vi "CompressAndUpdate(Enum).vi"(7 "force CVT update (false)":bool, 8 "error in":errorcluster, 9 "precision (6)":i16=6, 10 "enum variant":variant, 11 "command or variable name":string) -> (0 "error out":errorcluster)   [LabVIEW 2011]
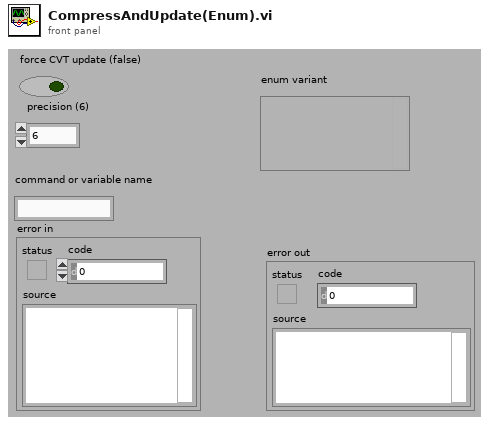
[diagram p1: front panel]
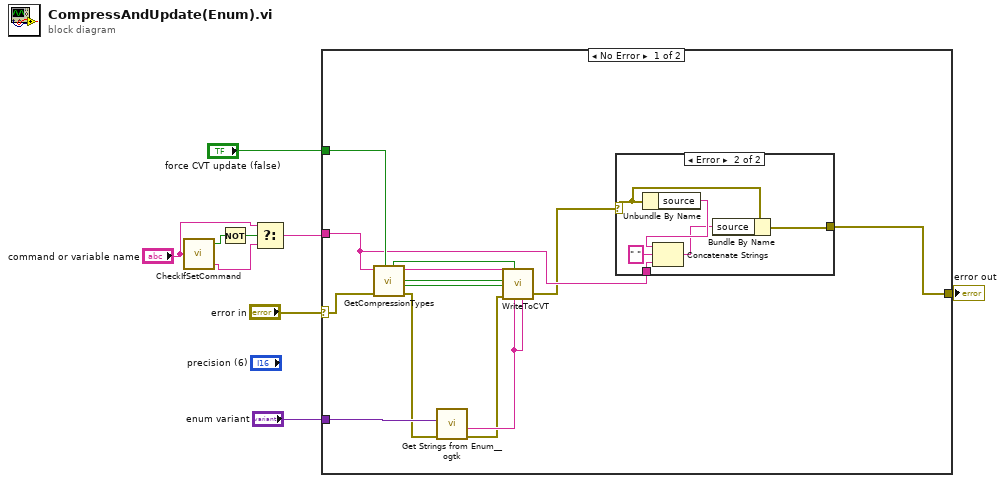
[diagram p0: block diagram]
diagram:
  n1 = call "CheckIfSetCommand.vi"("Command"="command or variable name") -> ("setCommand?"=w7:bool, "variable"=w4:string)  [unwired: 1 out]
  n2 = Not(x=w7) -> (.not. x?=w6:bool)
  n3 = Select(t="command or variable name", s=w6, f=w4) -> (s? t:f=w3:string)
  n4 = case shown="No Error" "error in" {
    selector: "error in" -> [w21 w30]
    tunnel: w3 -> [w12 _]
    tunnel: [w10 w30] -> w8
    tunnel: "force CVT update (false)" -> [w13 _]
    tunnel: "enum variant" -> [w22 _]
    frame No Error {
      n5 = call "GetCompressionTypes.vi"("force CVT update"=w13, "error in"=w21, "variable"=w12) -> ("error out"=w15:errorcluster, "non compressed"=w17:bool, "compressed"=w18:bool, "variable out"=w19:string, "force CVT update out"=w14:bool)  [unwired: 4 in]
      n6 = call "Get Strings from Enum__ogtk.vi"("error in (no error)"=w15, "Enum"=w22) -> ("error out"=w16:errorcluster, "String Value"=w20:string)  [unwired: 6 in, 2 out]
      n7 = call "WriteToCVT.vi"("non compressed string"=w20, "compressed string"=w20, "force CVT update"=w14, "error in"=w16, "non compressed"=w17, "compressed"=w18, "variable"=w19) -> ("error out"=w11:errorcluster)  [unwired: 4 in]
      n8 = case shown="Error" w11 {
        selector: w11 -> [w23 w26]
        tunnel: w12 -> [_ w28]
        tunnel: [w23 w24] -> w10
        frame No Error {
        }
        frame Error {
          n9 = Unbundle By Name(w26) -> ("source"=w27:string)
          n10 = Concatenate Strings(w27, " " ("string"), w28) -> (w25:string)
          n11 = Bundle By Name(cluster=w26, "source"=w25) -> (w24:errorcluster)
        }
      }
    }
    frame Error {
    }
  }
  "error out" <- w8
